vi "sub_pkt_generate.vi"(8 "accesscode (bit)":i8[](array[numeric]), 11 "byte stream":u8[](array[numeric])) -> (3 "bit pkt":i16[](array[numeric]))   [LabVIEW 2014]
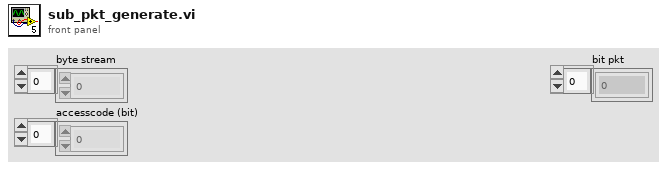
[diagram p1: front panel]
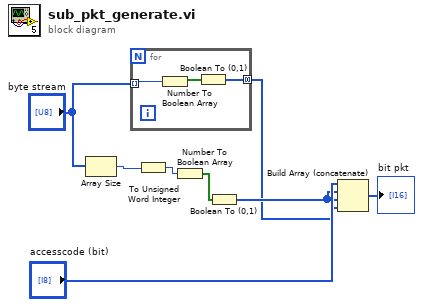
[diagram p0: block diagram]
diagram:
  n1 = Array Size(array="byte stream") -> (size(s)=w8:i32)
  n2 = for {
    tunnel: "byte stream" -> [w11] mode=indexing
    tunnel: [w9] -> w2 mode=concatenating
    n3 = Number To Boolean Array(number=w11) -> (Boolean array=w10:bool[])
    n4 = Boolean To (0,1)(Boolean=w10) -> (0, 1=w9:i16[])
  }
  n5 = To Unsigned Word Integer(number=w8) -> (unsigned 16bit integer=w6:u16)
  n6 = Number To Boolean Array(number=w6) -> (Boolean array=w5:bool[])
  n7 = Boolean To (0,1)(Boolean=w5) -> (0, 1=w4:i16[])
  n8 = Build Array (concatenate)("accesscode (bit)", w4, w4, w2) -> (→"bit pkt":i16[])
